vi "Set configuration chain.vi"(8 "error in (no error)":errorcluster, 9 "class names":string[](array[string]), 10 "configuration":variant[](array[variant]), 11 "focus in":refnum<class "focus.lvclass">) -> (0 "error out":errorcluster, 3 "focus out":refnum<class "focus.lvclass">)   [LabVIEW 2012, in "focus.lvclass"]
uses:
  focus.lvclass
  <vilib>/Distrio/Murmex/Murmex/Murmex.lvclass
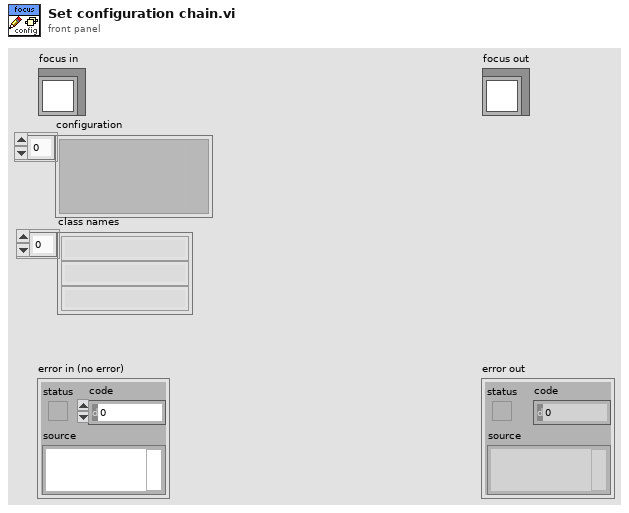
[diagram p1: front panel]
types:
  T1 = typedef "focus.lvclass/configuration_cluster.ctl" = cluster{"Port":T2, "Baudrate":T3, "update frequency":dbl[unit], "S/N Master controller":string, "Interface":T4, "soft limit min":dbl, "soft limit max":dbl, "startup speed":dbl[unit]}
  T2 = typedef "focus.lvclass/port_focus.ctl" = i32
  T3 = typedef "focus.lvclass/baud_rate_focus.ctl" = u16
  T4 = typedef "focus.lvclass/connection_type_focus.ctl" = enum16{"RS232", "RS232 DaisyChain", "USB", "USB_DaisyChain"}
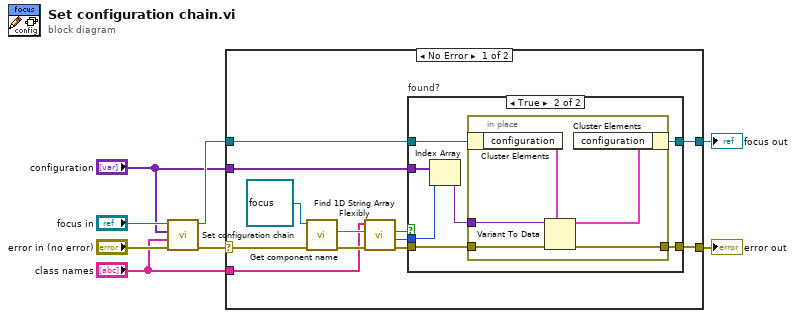
[diagram p0: block diagram]
diagram:
  n1 = call-parent "Set configuration chain.vi"("error in (no error)"="error in (no error)", "class names"="class names", "configuration"="configuration", "Murmex in"="focus in") -> ("error out"=w6:errorcluster, "Murmex out"=w5:refnum<class "focus.lvclass">)  [unwired: 6 in]
  n2 = case shown="No Error" w6 {
    selector: w6 -> [w18 w35]
    tunnel: w5 -> [w16 w36]
    tunnel: "configuration" -> [w15 _]
    tunnel: "class names" -> [w14 _]
    tunnel: [w9 w35] -> w2
    tunnel: [w10 w36] -> w1
    frame No Error {
      n3 = call <vilib>:"Get component name.vi"("error in (no error)"=w18, "Murmex in"=refnum<class "focus.lvclass"> refnum ("focus")) -> ("error out"=w20:errorcluster, "component name"=w19:string)  [unwired: 7 in, 1 out]
      n4 = call <vilib>:"Find 1D String Array Flexibly.vi"("error in (no error)"=w20, "element"=w19, "array"=w14) -> ("error out"=w13:errorcluster, "index of element"=w12:i32, "found?"=w11:bool)  [unwired: 6 in]
      n5 = case "found?" shown="True" w11 {
        tunnel: w12 -> [_ w27]
        tunnel: w13 -> [w22 w26]
        tunnel: [w22 w25] -> w9
        tunnel: [w21 w23] -> w10
        tunnel: w16 -> [w21 w29]
        tunnel: w15 -> [_ w28]
        frame False {
        }
        frame True {
          n6 = Index Array(array=w28, index=w27) -> (element=w24:variant)
          n7 = in-place {
            in-place-border: w26 -> [w34]
            in-place-border: [w33] -> w25
            in-place-border: w24 -> [w30]
            n8 = in-place-cluster #1(w29) -> ("configuration"=w32:T1)
            n9 = Variant To Data(error in=w34, type=w32, Variant=w30) -> (data=w31:T1, error out=w33:errorcluster)
            n10 = in-place-cluster #1("configuration"=w31) -> (w23:refnum<class "focus.lvclass">)
          }
        }
      }
    }
    frame Error {
    }
  }
  "error out" <- w2
  "focus out" <- w1
